vi "RampPower.vi"() -> ()   [LabVIEW 2017]
panel:
  in  "Delay":dbl
  out "Old Power":dbl
  in  "Factor":dbl
  out "Power":dbl
  in  "Joystick value":dbl step=0.1
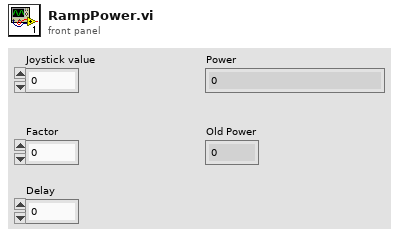
[diagram p1: front panel]
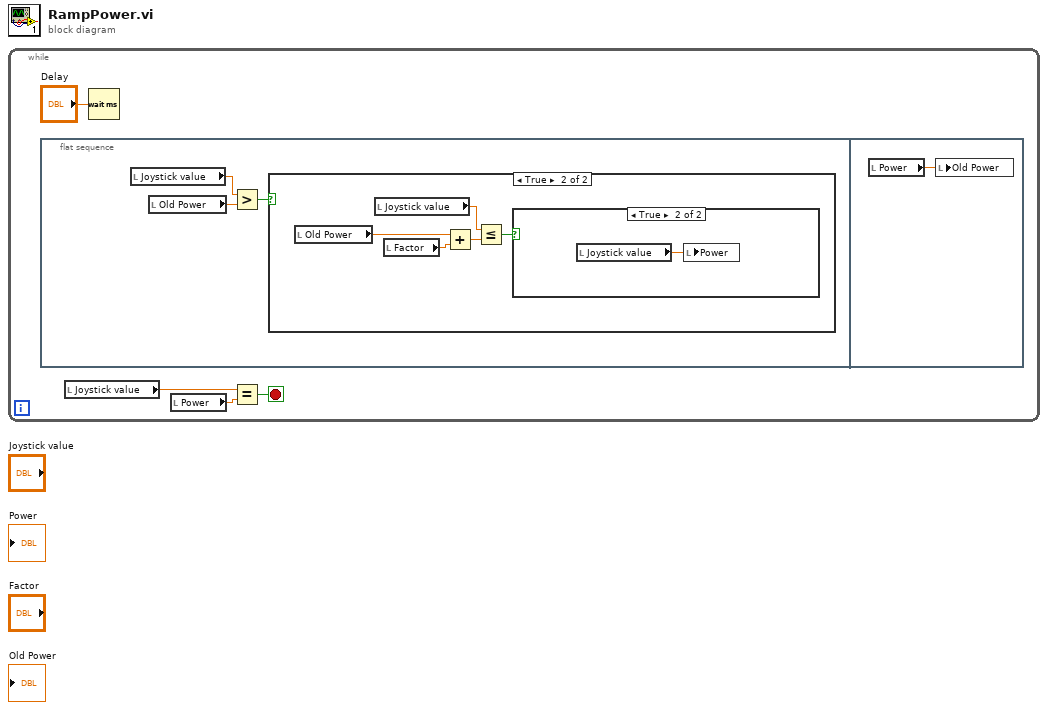
[diagram p0: block diagram]
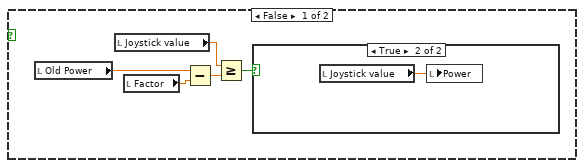
[diagram p2: hidden frame]
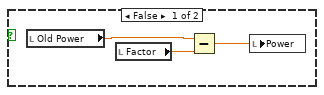
[diagram p3: hidden frame]
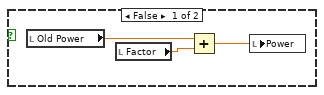
[diagram p4: hidden frame]
diagram:
  n1 = while {
    stop <- w4 stop-if-true
    n2 = flat-sequence {
      frame #0 {
        n3 = local read "Joystick value"() -> (w7:dbl)
        n4 = local read "Old Power"() -> (w6:dbl)
        n5 = Greater?(x=w7, y=w6) -> (0:w5:bool)
        n6 = case shown="True" w5 {
          frame False {
            n7 = local read "Old Power"() -> (w11:dbl)
            n8 = local read "Joystick value"() -> (w12:dbl)
            n9 = local read "Factor"() -> (w10:dbl)
            n10 = Subtract(x=w11, y=w10) -> (x-y=w9:dbl)
            n11 = Greater Or Equal?(x=w12, y=w9) -> (x >= y?=w8:bool)
            n12 = case shown="True" w8 {
              frame False {
                n13 = local read "Old Power"() -> (w15:dbl)
                n14 = local read "Factor"() -> (w14:dbl)
                n15 = Subtract(x=w15, y=w14) -> (x-y=w13:dbl)
                n16 = local write "Power"(w13) -> ()
              }
              frame True {
                n17 = local read "Joystick value"() -> (w16:dbl)
                n18 = local write "Power"(w16) -> ()
              }
            }
          }
          frame True {
            n19 = local read "Old Power"() -> (w20:dbl)
            n20 = local read "Joystick value"() -> (w21:dbl)
            n21 = local read "Factor"() -> (w19:dbl)
            n22 = Add(x=w20, y=w19) -> (x+y=w18:dbl)
            n23 = Less Or Equal?(x=w21, y=w18) -> (x <= y?=w17:bool)
            n24 = case shown="True" w17 {
              frame False {
                n25 = local read "Old Power"() -> (w23:dbl)
                n26 = local read "Factor"() -> (w24:dbl)
                n27 = Add(x=w23, y=w24) -> (x+y=w22:dbl)
                n28 = local write "Power"(w22) -> ()
              }
              frame True {
                n29 = local read "Joystick value"() -> (w25:dbl)
                n30 = local write "Power"(w25) -> ()
              }
            }
          }
        }
      }
      frame #1 {
        n31 = local read "Power"() -> (w26:dbl)
        n32 = local write "Old Power"(w26) -> ()
      }
    }
    n33 = local read "Joystick value"() -> (w3:dbl)
    n34 = Wait (ms)(milliseconds to wait="Delay") -> ()  [unwired: 1 out]
    n35 = local read "Power"() -> (w2:dbl)
    n36 = Equal?(x=w3, y=w2) -> (x = y?=w4:bool)
  }
